vi "Open-file.vi"(8 "error in (no error)":errorcluster, 10 "Full path":path, 11 "SettingsFile in":refnum<class "SettingsFile.lvclass">) -> (0 "error out":errorcluster, 2 "File reference":refnum<file>, 3 "SettingsFile out":refnum<class "SettingsFile.lvclass">)   [LabVIEW 2013, in "SettingsFile.lvlib" / "SettingsFile.lvclass"]
uses:
  SettingsFile.lvclass
  SettingsFile.lvclass/SettingsFile.ctl
  Errors.ctl
  <vilib>/Utility/config.llb/NI_LVConfig.lvlib
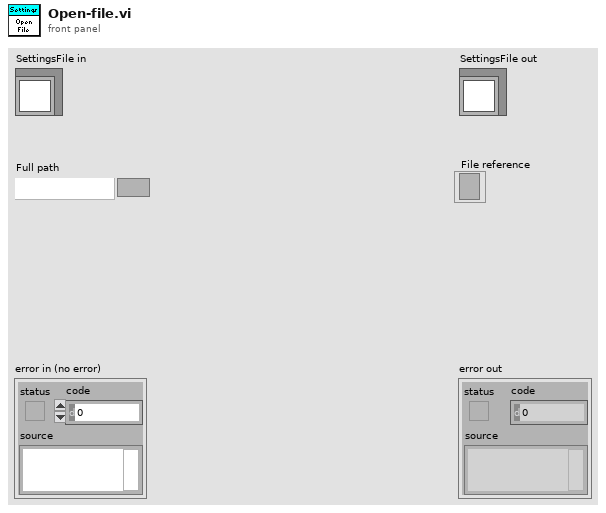
[diagram p1: front panel]
types:
  T1 = typedef "SettingsFile.lvlib/SettingsFile.lvclass/Errors.ctl" = enum16{"Not implemented", "Command not recognized", "Invalid input", "No connection", "Timeout", "Invalid file type", "No file access"}
  T2 = enum16{"open", "replace", "create", "open or create", "replace or create", "replace or create with confirmation"}
  T3 = typedef "NI_LVConfig.lvlib/Config Data RefNum.ctl" = refnum<k1>
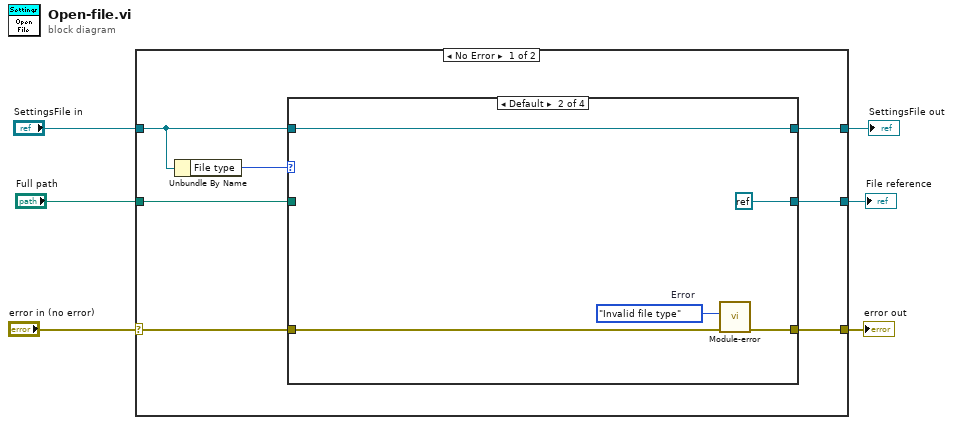
[diagram p0: block diagram]
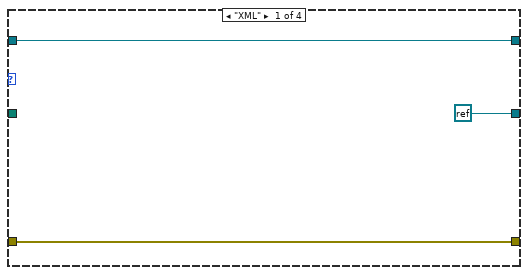
[diagram p2: hidden frame]
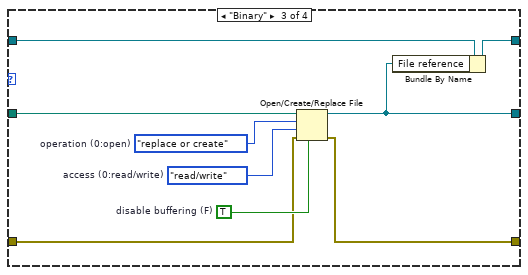
[diagram p3: hidden frame]
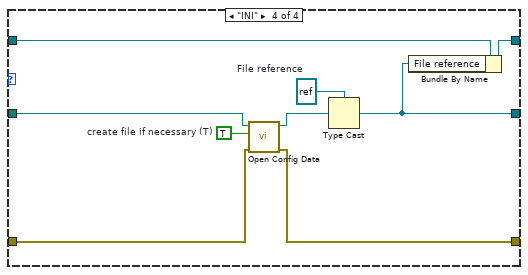
[diagram p4: hidden frame]
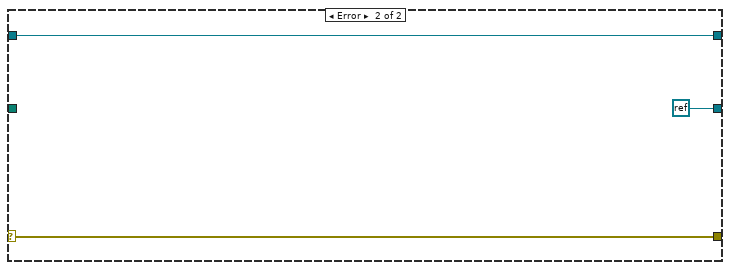
[diagram p5: hidden frame]
diagram:
  n1 = case shown="No Error" "error in (no error)" {
    selector: "error in (no error)" -> [w12 w42]
    tunnel: [w11 w42] -> w5
    tunnel: [w10 w41] -> w3
    tunnel: "SettingsFile in" -> [w8 w41]
    tunnel: "Full path" -> [w13 _]
    tunnel: [w9 refnum<k0> refnum] -> w1
    frame No Error {
      n2 = Unbundle By Name(w8) -> ("File type"=w7:enum16{"XML", "INI", "Binary"})
      n3 = case shown="Default" w7 {
        tunnel: w8 -> [w16 w21 w30 w39]
        tunnel: w13 -> [_ _ w29 w38]
        tunnel: w12 -> [w14 w18 w25 w35]
        tunnel: [w14 w19 w24 w34] -> w11
        tunnel: [w16 w21 w23 w32] -> w10
        tunnel: [refnum<k0> refnum refnum<k0> refnum w22 w31] -> w9
        frame "XML" {
        }
        frame Default {
          w17 = Errors."Invalid file type"  # Error
          n4 = call "Module-error.vi"("error in (no error)"=w18, "Error"=w17) -> ("error out"=w19:errorcluster)  [unwired: 9 in]
        }
        frame "Binary" {
          w26 = TRUE  # disable buffering (F)
          w27 = enum16{"read/write", "read-only", "write-only"}."read/write"  # access (0:read/write)
          w28 = T2."replace or create"  # operation (0:open)
          n5 = Open/Create/Replace File(file path (use dialog)=w29, error in=w25, operation (0:open)=w28, access (0:read/write)=w27, disable buffering (F)=w26) -> (refnum out=w22:refnum<file>, error out=w24:errorcluster)  [unwired: 1 in, 1 out]
          n6 = Bundle By Name(cluster=w30, "File reference"=w22) -> (w23:refnum<class "SettingsFile.lvclass">)
        }
        frame "INI" {
          w33 = TRUE  # create file if necessary (T)
          w36 = refnum<file> refnum  # File reference
          n7 = call <vilib>:"Open Config Data.vi"("error in (no error)"=w35, "create file if necessary (T)"=w33, "configuration file path"=w38) -> ("error out"=w34:errorcluster, "refnum"=w37:T3)  [unwired: 6 in, 1 out]
          n8 = Type Cast(type=w36, x=w37) -> (*(type *) &x=w31:refnum<file>)
          n9 = Bundle By Name(cluster=w39, "File reference"=w31) -> (w32:refnum<class "SettingsFile.lvclass">)
        }
      }
    }
    frame Error {
    }
  }
  "error out" <- w5
  "SettingsFile out" <- w3
  "File reference" <- w1
